vi "Formula Methods.vi"() -> ()   [LabVIEW 2019]
uses:
  <vilib>/express/express arith-compare/Formula/XNode/ExpressFormulaBlockNode.xnode
panel:
  in  "UI":enum32{"Question 1", "Question 2"}(tab)
  out "V M3":dbl
  out "V M2":dbl
  out "V M1":dbl
  out "SA M3":dbl
  out "SA M2":dbl
  out "SA M1":dbl
  in  "Height":dbl
  in  "Radius":dbl
  # "Volume"
  # "Surface Area"
  # "Inputs"
  # "2xy^2 + 4xy + 8"
  # "Implement the 3 methods as shown in the previous example."
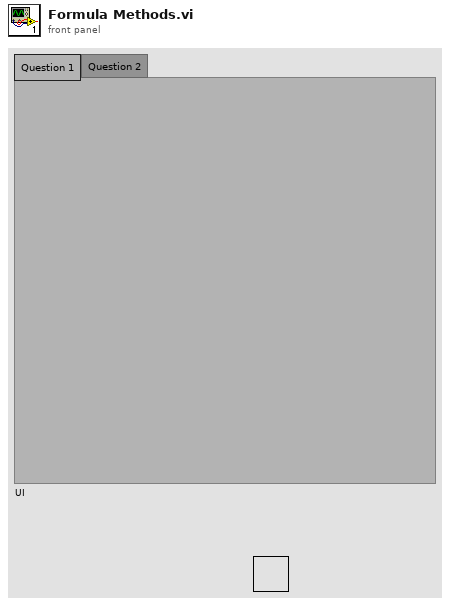
[diagram p1: front panel]
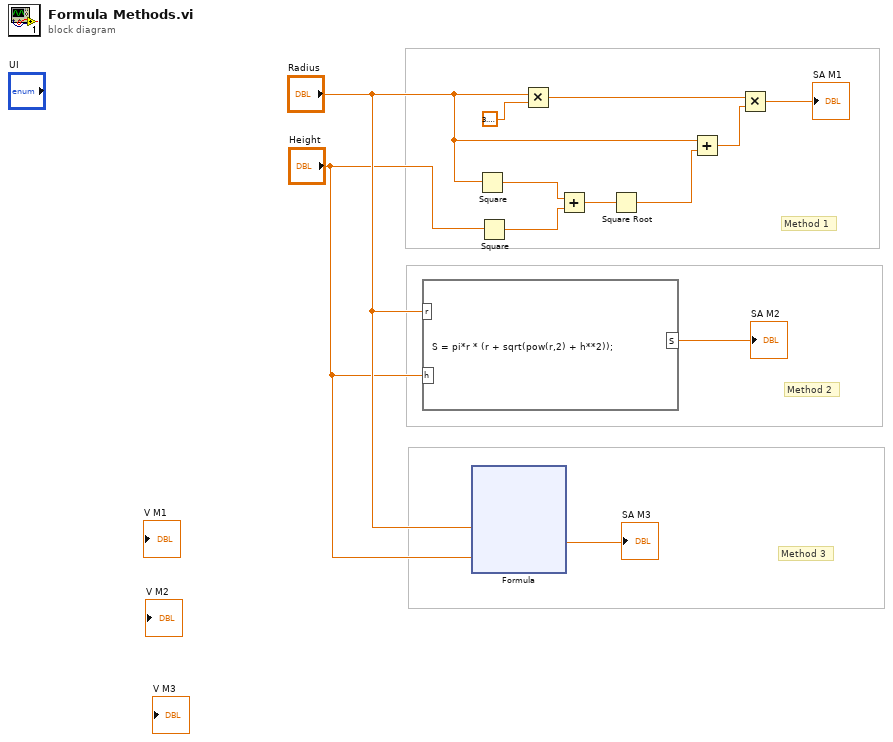
[diagram p0: block diagram]
diagram:
  # "Method 3"
  # "Method 2"
  # "Method 1"
  n1 = formula code="S = pi*r * (r + sqrt(pow(r,2) + h**2));"("r"="Radius", "h"="Height") -> ("S"=→"SA M2":dbl)
  n2 = xnode "Formula"("r"="Radius", "h"="Height") -> ("Result"=→"SA M3":dbl)  [unwired: 1 in, 1 out]
  n3 = Square(x="Radius") -> (x^2=w11:dbl)
  n4 = Square(x="Height") -> (x^2=w10:dbl)
  n5 = Multiply(x="Radius", y=3.141592653589793) -> (x*y=w7:dbl)
  n6 = Add(x=w11, y=w10) -> (x+y=w9:dbl)
  n7 = Square Root(x=w9) -> (sqrt(x)=w8:dbl)
  n8 = Add(x="Radius", y=w8) -> (x+y=w6:dbl)
  n9 = Multiply(x=w7, y=w6) -> (x*y=→"SA M1":dbl)
